vi "Project Euler Problem 2 Solution.vi"() -> ()   [LabVIEW 2017]
panel:
  out "?":i32
  out "?":i32
  # "Problem Description:\n\nBy considering the terms in the Fibonacci sequence whose values do not exceed four million, find the sum of the even-valued terms."
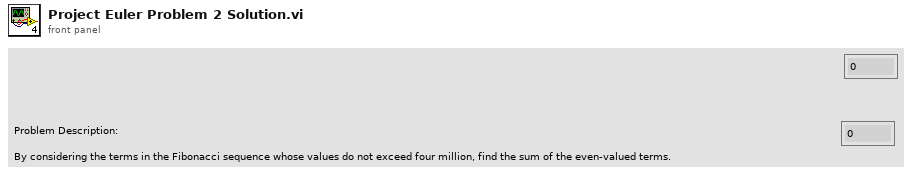
[diagram p1: front panel]
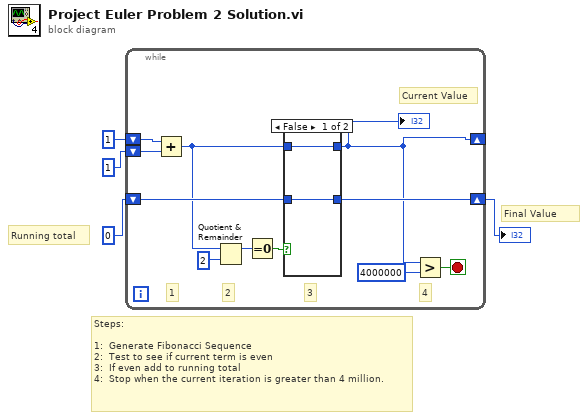
[diagram p0: block diagram]
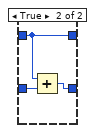
[diagram p2: hidden frame]
diagram:
  # "Final Value"
  # "Running total"
  # "Steps:\n\n1:  Generate Fibonacci Sequence\n2:  Test to see if current term is even\n3:  If even add to running total\n4:  Stop when the current iteration is greater than 4 million."
  n1 = while {
    shift-right: [w7] -> _
    shift-left: 1 -> [w15]
    shift-left: 1 -> [w14]
    shift-right: [w8] -> w1
    shift-left: 0 -> [w10]
    stop <- w5 stop-if-true
    # "4"
    # "3"
    # "2"
    # "1"
    # "Current Value"
    n2 = Add(x=w15, y=w14) -> (x+y=w9:i32)
    n3 = Quotient & Remainder(x=w9, y=2) -> (x-y*floor(x/y)=w12:i32)  [unwired: 1 out]
    n4 = Equal To 0?(x=w12) -> (x = 0?=w11:bool)
    n5 = case shown="False" w11 {
      tunnel: w10 -> [w16 w20]
      tunnel: w9 -> [w17 w19]
      tunnel: [w17 w19] -> w7
      tunnel: [w16 w18] -> w8
      frame False {
      }
      frame True {
        n6 = Add(x=w19, y=w20) -> (x+y=w18:i32)
      }
    }
    "?" <- w7
    n7 = Greater?(x=w7, y=4000000) -> (0:w5:bool)
  }
  "?" <- w1
